vi "Create xls File.vi"(4 "error in":errorcluster) -> (0 "error out":errorcluster, 1 "Valid File":bool, 2 "path":path, 3 "refnum":refnum<file>)   [LabVIEW 2015]
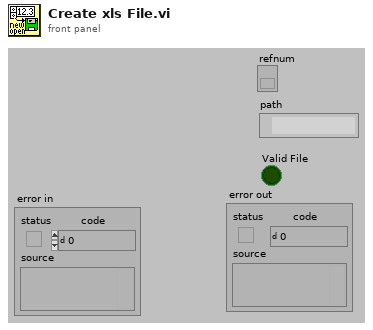
[diagram p1: front panel]
types:
  T1 = enum16{"open", "open or create", "create or replace", "create", "open (read only)"}
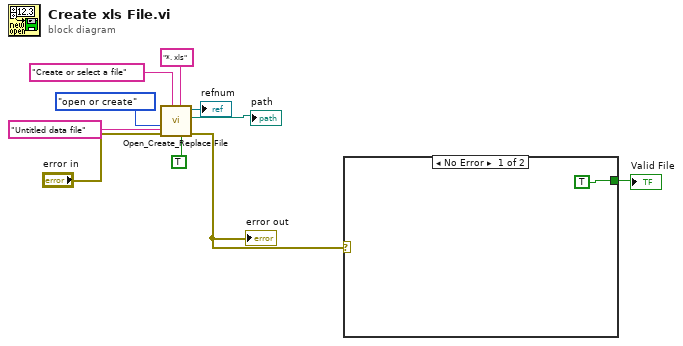
[diagram p0: block diagram]
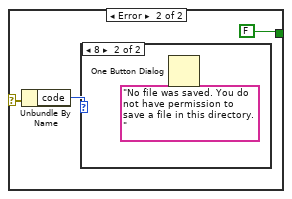
[diagram p2: hidden frame]
diagram:
  n1 = call <vilib>:"Open_Create_Replace File.vi"("advisory dialog? (display:T)"=TRUE, "pattern"="*. xls", "default name"="Untitled data file", "prompt"="Create or select a file", "error in (no error)"="error in", "function (open:0)"=T1."open or create") -> ("error out"=w4:errorcluster, "new file path"=→"path":path, "refnum"=→"refnum":refnum<file>)  [unwired: 2 in, 1 out]
  "error out" <- w4
  n2 = case shown="No Error" w4 {
    selector: w4 -> [_ w14]
    tunnel: [TRUE ("Valid File") FALSE ("Valid File")] -> w1
    frame No Error {
    }
    frame Error {
      n3 = Unbundle By Name(w14) -> ("code"=w13:i32)
      n4 = case shown="8" w13 {
        frame 0, Default {
        }
        frame 8 {
          n5 = One Button Dialog(message="No file was saved. You do not have permission to save a file in this directory.") -> ()  [unwired: 1 in, 1 out]
        }
      }
    }
  }
  "Valid File" <- w1
